vi "p1.vi"() -> ()   [LabVIEW 2021, in "d13.lvlib"]
uses:
  d13.lvlib
  AOC/AOC.lvlib
panel:
  in  "Example":string="[1,1,3,1,1]\n[1,1,5,1,1]\n\n[[1],[2,3,4]]\n[[1],4]\n\n[9]\n[[8,7,6]]\n\n[[4,4],4,4]\n[[4,4],4,4,4]\n\n[7,7,7,7]\n[7,7,7]\n\n[]\n[3]\n\n[[[]]]\n[[]]\n\n[1,[2,[3,[4,[5,6,7]]]],8,9]\n[1,[2,[3,[4,[5,6,0]]]],8,9]"
  in  "Example":bool
  out "Answer":i64=5675
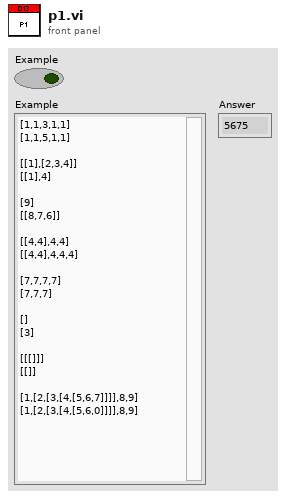
[diagram p1: front panel]
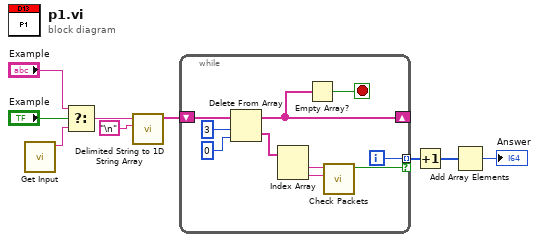
[diagram p0: block diagram]
diagram:
  n1 = call "Get Input.vi"() -> ("Input"=w9:string)  [unwired: 11 in]
  n2 = Select(t="Example", s="Example", f=w9) -> (s? t:f=w8:string)
  n3 = call <vilib>:"Delimited String to 1D String Array.vi"("delimiter"="\n", "delimited string"=w8) -> ("string array"=w4:string[])  [unwired: 9 in]
  n4 = while {
    tunnel: [w15] -> w3 mode=indexing if=w10
    shift-right: [w13] -> _
    shift-left: w4 -> [w19]
    i -> [w15]
    stop <- w17 stop-if-true
    n5 = Delete From Array(array=w19, length=3 ("y"), index=0) -> (deleted portion=w16:string[], array with subset deleted=w13:string[])
    n6 = Index Array(array=w16) -> (element #1=w12:string, element #2=w11:string)  [unwired: 2 in]
    n7 = Empty Array?(array=w13) -> (empty?=w17:bool)
    n8 = call "Check Packets.vi"("Right Packet"=w11, "Left Packet"=w12) -> ("Correct Order?"=w10:bool)  [unwired: 8 in, 1 out]
  }
  n9 = Increment(x=w3) -> (x+1=w2:i32[])
  n10 = Add Array Elements(numeric array=w2) -> (sum=→"Answer":i32)
